vi "System.vi"() -> ()   [LabVIEW 2023]
panel:
  in  "Stop":bool
  out "Waveform Chart - Temperatures":T1(graph)
  out "Waveform Chart - Control Signal":dbl(graph)
  out "T_real":dbl=29.097264063224614
  out "Temp [C]":dbl=29.659641078261295
  out "Error Term":dbl
  in  "Tab Control":T2(tab)=enum."Model params"
  in  "Time Step [s]":dbl=0.1
  in  "MA Filter":bool
  out "Control Signal [V]":dbl format="%#_2g"
  in  "Desired Temperature [deg C]":dbl(slide)=30.0 scale=20.0..40.0
  in  "Air Heater Params":T3={"Temp_init [C]"=22.0, "K [C/V]"=3.2, "theta_t [s]"=5.5, "theta_d [s]"=3.0, "theta_d_out_init [V]"=0.0, "theta_d_max [s]"=5.0}
  in  "Temp Environment [C]":dbl(slide)=22.0 scale=0.0..35.0
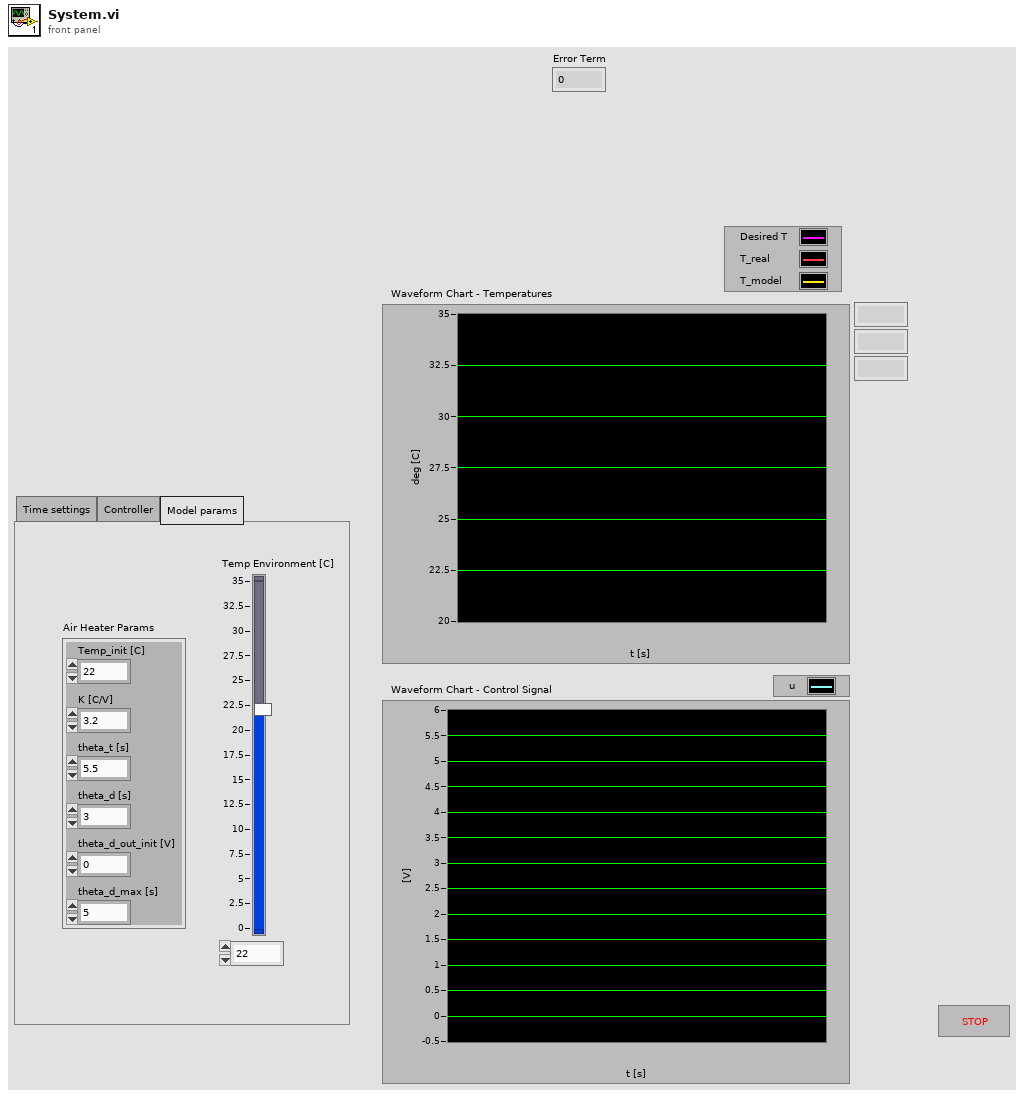
[diagram p1: front panel]
types:
  T1 = cluster{"r [deg C]":dbl, "T_real":dbl, "T_real":dbl}
  T2 = enum32{"Time settings", "Controller", "Model params"}
  T3 = cluster{"Temp_init [C]":dbl, "K [C/V]":dbl, "theta_t [s]":dbl, "theta_d [s]":dbl, "theta_d_out_init [V]":dbl, "theta_d_max [s]":dbl}
  T4 = cluster{"r [deg C]":dbl, "T_real":dbl, "T_real":dbl}[]
  T5 = cluster{"Desired Temperature [deg C]":dbl, "T_real":dbl, "Temp [C]":dbl}
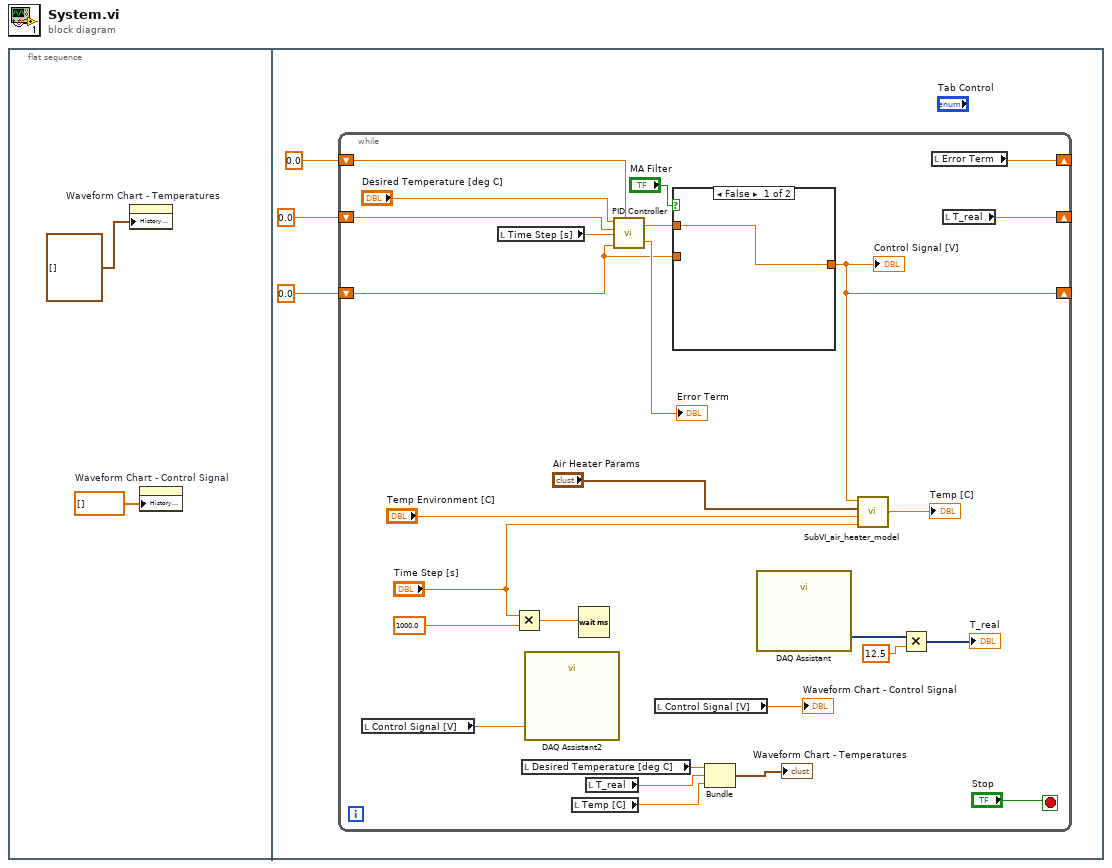
[diagram p0: block diagram]
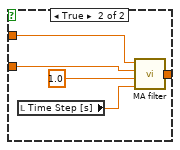
[diagram p2: hidden frame]
diagram:
  n1 = flat-sequence {
    frame #0 {
      n2 = property on="Waveform Chart - Temperatures" class="WFChart (strict)"("History Data"=T4 []) -> ()  [unwired: 2 in, 2 out]
      n3 = property on="Waveform Chart - Control Signal" class="WFChart (strict)"("History Data"=dbl[] []) -> ()  [unwired: 2 in, 2 out]
    }
    frame #1 {
      n4 = while {
        shift-right: [w7] -> _
        shift-left: 0.0 ("ui_1") -> [w9]
        shift-right: [w22] -> _
        shift-left: 0.0 ("Temp [C]") -> [w17]
        shift-right: [w13] -> _
        shift-left: 0.0 -> [w12]
        stop <- "Stop" stop-if-true
        n5 = local read "Control Signal [V]"() -> (w11:dbl)
        n6 = local read "Time Step [s]"() -> (w15:dbl)
        n7 = Multiply(x="Time Step [s]", y=1000.0) -> (x*y=w31:dbl)
        n8 = local read "Desired Temperature [deg C]"() -> (w27:dbl)
        n9 = call "DAQ Assistant2"("data"=w11) -> ()  [unwired: 17 in, 2 out]
        n10 = local read "Temp [C]"() -> (w19:dbl)
        n11 = Wait (ms)(milliseconds to wait=w31) -> ()  [unwired: 1 out]
        n12 = local read "T_real"() -> (w20:dbl)
        n13 = call "PID Controller.vi"("Reference Value"="Desired Temperature [deg C]", "Process Value"=w17, "Time step [s]"=w15, "Previous signal"=w9, "Previous error"=w12) -> ("Process signal"=w8:dbl, "Error Term"=→"Error Term":dbl)
        n14 = local read "Control Signal [V]"() -> (→"Waveform Chart - Control Signal":dbl)
        n15 = case shown="False" "MA Filter" {
          tunnel: w9 -> [_ w36]
          tunnel: w8 -> [w33 w35]
          tunnel: [w33 w34] -> w7
          frame False {
          }
          frame True {
            n16 = local read "Time Step [s]"() -> (w38:dbl)
            n17 = call "MA filter.vi"("dt"=w38, "Tw"=1.0, "y_1"=w36, "y"=w35) -> ("yf"=w34:dbl)
          }
        }
        "Control Signal [V]" <- w7
        n18 = Bundle("Desired Temperature [deg C]"=w27, "T_real"=w20, "Temp [C]"=w19) -> (→"Waveform Chart - Temperatures":T5)  [unwired: 1 in]
        n19 = call "DAQ Assistant"() -> ("data"=w25:dynamicdata)  [unwired: 17 in, 2 out]
        n20 = call "SubVI_air_heater_model.vi"("T_step [s]"="Time Step [s]", "Temp_env [C]"="Temp Environment [C]", "Cluster_air_heater_params"="Air Heater Params", "u [V]"=w7) -> ("Temp [C]"=→"Temp [C]":dbl)
        n21 = Multiply(x=w25, y=12.5) -> (x*y=→"T_real":dynamicdata)
        n22 = local read "Error Term"() -> (w13:dbl)
        n23 = local read "T_real"() -> (w22:dbl)
      }
    }
  }
